vi "Plotmatrix Appearance Property.vi"(6 "Update?":bool, 8 "error in (no error)":errorcluster, 9 "Palette Visible":T1, 11 "Single XY Plot In":refnum<vi>) -> (0 "error out":errorcluster, 3 "Single XY Plot Out":refnum<vi>)   [LabVIEW 2017, in "XY Plot Matrix.lvclass"]
uses:
  <vilib>/Math Plots/2D Math Plots/XY Plot Matrix/XY Plot Matrix/XY Plot Matrix.lvclass
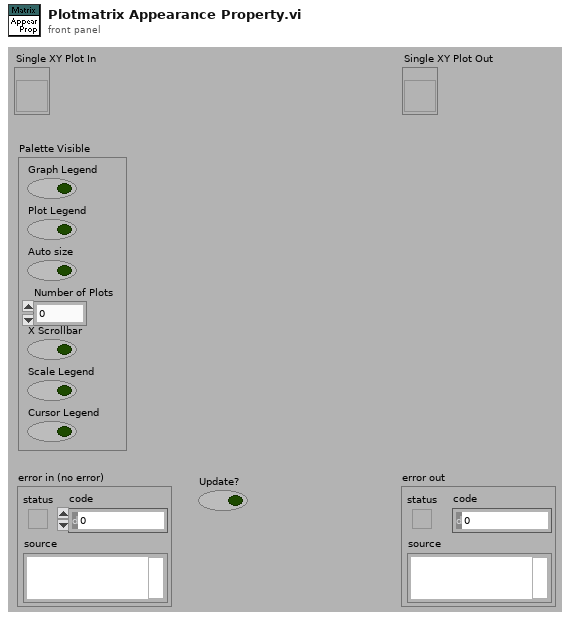
[diagram p1: front panel]
types:
  T1 = cluster{"Graph Legend":bool, "Plot Legend":bool, "Auto size":bool, "Number of Plots":u32, "X Scrollbar":bool, "Scale Legend":bool, "Cursor Legend":bool}
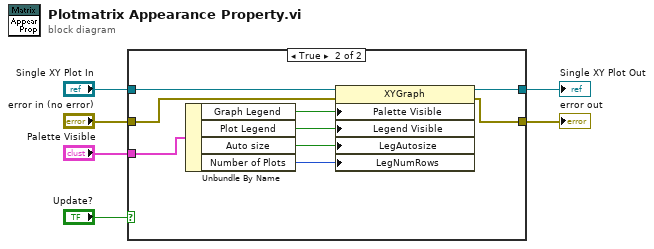
[diagram p0: block diagram]
diagram:
  n1 = case shown="True" "Update?" {
    tunnel: [w7 w17] -> w2
    tunnel: "error in (no error)" -> [w7 w16]
    tunnel: [w8 w15] -> w4
    tunnel: "Single XY Plot In" -> [w8 w14]
    tunnel: "Palette Visible" -> [_ w13]
    frame False {
    }
    frame True {
      n2 = Unbundle By Name(w13) -> ("Graph Legend"=w12:bool, "Plot Legend"=w11:bool, "Auto size"=w10:bool, "Number of Plots"=w9:u32)
      n3 = property class="XYGraph"(reference=w14, error in=w16, "Palette Visible"=w12, "Legend Visible"=w11, "LegAutosize"=w10, "LegNumRows"=w9) -> (reference out=w15:refnum<vi>, error out=w17:errorcluster)
    }
  }
  "Single XY Plot Out" <- w4
  "error out" <- w2
